vi "Read WiringRules[].vi"(11 "PolymorphicInstance in":refnum<class "PolymorphicInstance.lvclass">) -> (2 "WiringRules[]":T1(array[ring]), 3 "PolymorphicInstance out":refnum<class "PolymorphicInstance.lvclass">)   [LabVIEW 2013, in "PolymorphicInstance.lvclass"]
uses:
  PolymorphicInstance.lvclass
  PolymorphicInstance.lvclass/PolymorphicInstance.ctl
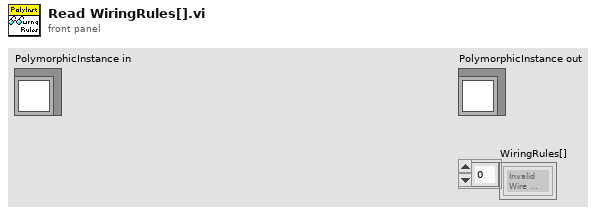
[diagram p1: front panel]
types:
  T1 = enum16{"Invalid Wire Rule", "Required", "Recommended", "Optional", "Dynamic Dispatch"}[]
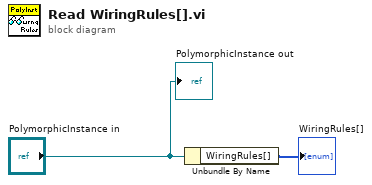
[diagram p0: block diagram]
diagram:
  n1 = Unbundle By Name("PolymorphicInstance in") -> ("WiringRules[]"=→"WiringRules[]":T1)
  "PolymorphicInstance out" <- "PolymorphicInstance in"
